vi "mainSC.vi"() -> ()   [LabVIEW 2021]
uses:
  <vilib>/Platform/TimedLoop/XDataNode/timing_clust.ctl
  <vilib>/Platform/TimedLoop/XDataNode/nitl_modes.ctl
  <vilib>/Platform/TimedLoop/XDataNode/wakeup.ctl
  <vilib>/xnet/xnet.llb/XNET Frame CAN.ctl
  <vilib>/xnet/xnet.llb/XNET Frame Type CAN.ctl
  <vilib>/xnet/xnet.llb/XNET Read (Frame CAN).vi
  <vilib>/xnet/xnet.llb/XNET Write (Frame CAN).vi
  <vilib>/Utility/error.llb/Error Cluster From Error Code.vi
  <vilib>/rvi/errors/niLvFpgaAdjustHostInterfaceError.vi
  General Purpose/FPGAref.ctl
  <vilib>/Platform/TimedLoop/XDataNode/XDataNode.xnode
  <vilib>/rvi/interface/nirviMethod/nirviMethod.xnode
  <vilib>/rvi/interface/nirviReadWriteControl/nirviReadWriteControl.xnode
  <vilib>/Platform/TimedLoop/XDataNode/XDNodeRunTimeDep.lvlib
  <vilib>/FPGAPlugInAG/Dynamic/niLvFpga_ReadFifo_Dynamic.vi
  <vilib>/rvi/errors/niLvFpgaMergeErrorWithErrorCode.vi
  NiFpgaLv.dll
  <vilib>/rvi/interface/Simulation/niFpgaSimulationCallBeginRW.vi
panel:
  out "IavFC":dbl
  out "TstackOut":dbl
  out "TstackIn":dbl
  out "FC_ph2":dbl
  out "ErrorBoolean":bool
  out "p_sp_max":dbl
  out "H2_flow":dbl
  in  "AnalogLoopPeriod(ms)":i64=250
  out "q_sp_min":dbl
  out "q_sp_max":dbl
  out "p_sp_min":dbl=2000.0
  out "Con_State 2":u8(ring) items=["Idle"=0, "Busy"=1, "Wait4srcON"=2, "Ready"=3, "VSC mode"=5, "CSC mode"=6, "Error"=9, "Wait4srcOFF"=10, "ISRC mode"=11, "VSRC mode"=12]
  out "ErrorListFCRaw":u8[](array[numeric])
  out "ErrorFC":bool=TRUE
  in  "Main Stop":bool
  in  "Isrc Mode":bool
  in  "Usr Demand":T1(ring)
  in  "Log Influx DB":bool=TRUE
  out "FCPS Voltage [V]":dbl
  out "FCPS Current [A]":dbl
  out "FC Power Setpoint":dbl
  out "Fuel Cell":T2 {"Tstack Out [degC]" format="%.3f"}
  out "Vdc DC Link":dbl
  out "Alarm list":string
  out "Error":u8(ring) items=["None", "Converter (water/temp/desat)", "Overvalue (hardware detected)", "Internal DC bus low", "Internal DC bus high", "External source DC low", "External source DC high", "Grid present (while VSC)", "Grid voltage out of range", "Grid frequency out of range", "No Grid (while CSC)", "Cannot clear (Manual clear needed)", "User Emergency"]
  in  "p_sp":dbl
  in  "q_sp":dbl
  in  "Shutdwn":bool
  in  "Clear":bool
  in  "SEND sp":bool
  in  "Start":bool
  in  "Emergency":bool
  in  "Meas":T3 {"Ia" format="%#.2f"; "Ib" format="%#.2f"; "Ic" format="%#.2f"; "Pa" format="%#.2f"; "Qa" format="%#.2f"; "Va" format="%#.2f"; "Pb" format="%#.2f"; "Qb" format="%#.2f"; "Vb" format="%#.2f"; "Pc" format="%#.2f"; "Qc" format="%#.2f"; "Vc" format="%#.2f"; "P" format="%#.2f"; "Q" format="%#.2f"; "S" format="%#.2f"; "PF" format="%#.2f"; "In" format="%#.2f"; "Vnpe" format="%#.2f"; "Vdc" format="%#.2f"; "Idc" format="%#.2f"; "Pdc" format="%#.2f"}
  out "DC":bool
  out "AC":bool
  out "CAN with Fuel Cell":bool
  out "V_src":dbl
  out "I_src":dbl
  out "Con_State":u8(ring) items=["Idle"=0, "Busy"=1, "Wait4srcON"=2, "Ready"=3, "VSC mode"=5, "CSC mode"=6, "Error"=9, "Wait4srcOFF"=10, "ISRC mode"=11, "VSRC mode"=12]
  in  "Conv CAN [ms]":i64=1
  out "Conv":T4
  out "CAN with Conv":bool
  in  "FC CAN [ms]":i64=50
  out "logging":bool
  in  "Meas [ms]":i64=10
  out "P":dbl format="%#.3f"
  out "Q":dbl format="%#.3f"
  out "S":dbl format="%#.3f"
  out "PF":dbl format="%#.3f"
  out "Measurements":bool
  # "FUEL CELL CONTROL"
  # "CONVERTER CONTROL"
  # "SETPOINTS"
  # "FUEL\nCELL"
  # "DC"
  # "AC"
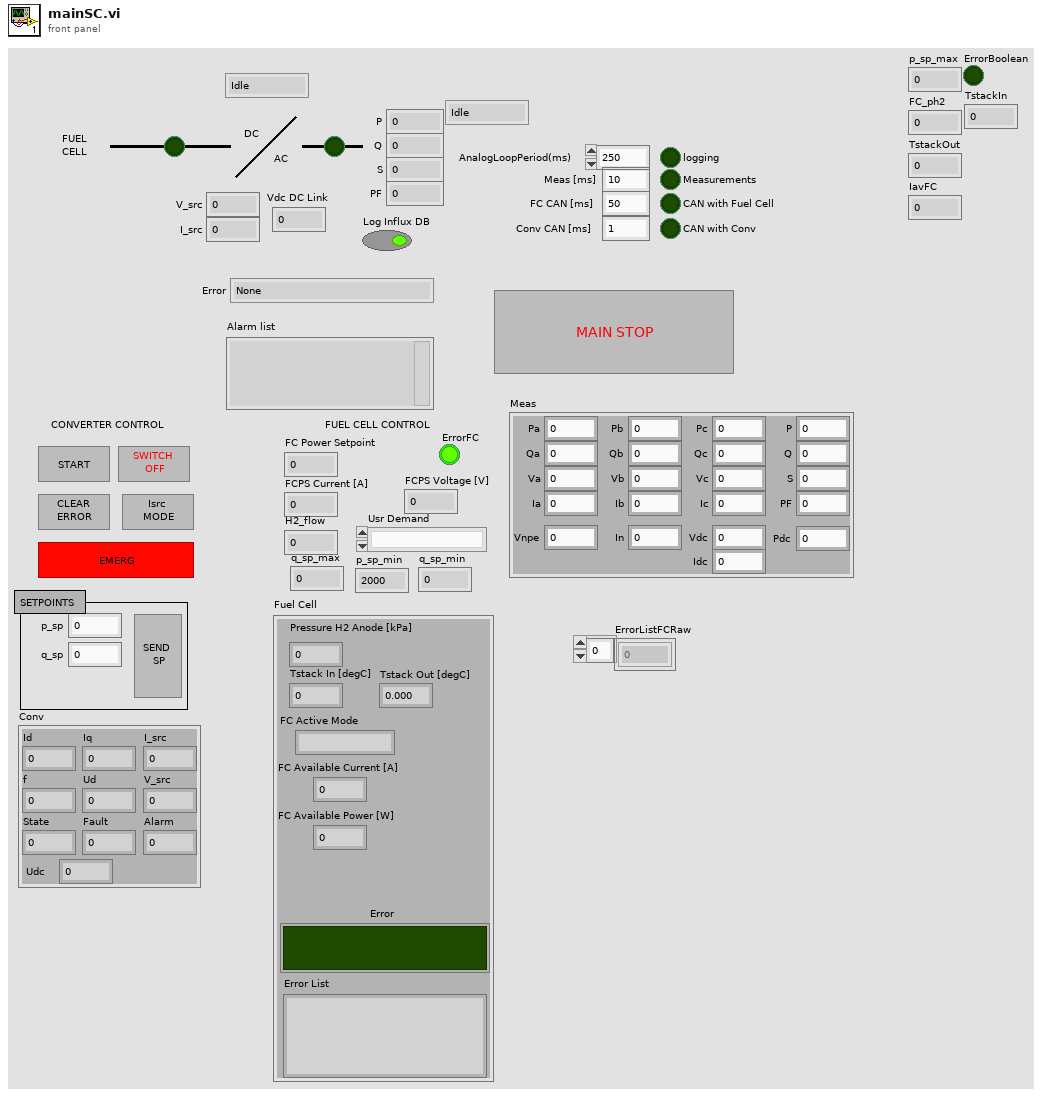
[diagram p1: front panel]
types:
  T1 = enum16{"", "Emergency Shut Down", "Shut Down", "Start"}
  T2 = cluster{"Tstack In [degC]":dbl, "Pressure H2 Anode [kPa]":dbl, "Tstack Out [degC]":dbl, "FC Available Current [A]":dbl, "FC Available Power [W]":dbl, "FC Active Mode":string, "Error":bool, "Error List":string}
  T3 = cluster{"Pa":dbl, "Qa":dbl, "Va":dbl, "Pb":dbl, "Qb":dbl, "Vb":dbl, "Pc":dbl, "Qc":dbl, "Vc":dbl, "P":dbl, "Q":dbl, "S":dbl, "PF":dbl, "In":dbl, "Vnpe":dbl, "Vdc":dbl, "Idc":dbl, "Pdc":dbl, "Ic":dbl, "Ib":dbl, "Ia":dbl}
  T4 = cluster{"Id":dbl, "Iq":dbl, "Ud":dbl, "f":dbl, "I_src":dbl, "V_src":dbl, "State":dbl, "Fault":dbl, "Alarm":dbl, "Udc":dbl}
  T5 = typedef "FPGAref.ctl" = refnum<k20>
  T6 = typedef "XDNodeRunTimeDep.lvlib/timing_clust.ctl" = cluster{"Expected End [f-1]":u64, "Actual End [f-1]":u64, "Finished Late? [f-1]":bool, "Expected End [i-1]":u64, "Actual End [i-1]":u64, "Finished Late? [i-1]":bool, "Expected Start [i]":u64, "Actual Start [i]":u64, "Expected Start [f]":u64, "Actual Start [f]":u64, "Source Name":string, "Structure Name":string, "Period":i64, "Deadline":i64, "Offset":i64, "Start":i64, "Priority":i32, "Timeout":i32, "Mode":T7, "Wakeup Reason":T8, "Error":errorcluster, "Source Type":string, "Secondary Source Type":string, "Global End Time":u64, "Global Start Time":u64, "Frame Duration":u64, "Iteration Duration":u64, "Assigned CPU":i32, "I/O Scan Engine Mode":u32}
  T7 = typedef "XDNodeRunTimeDep.lvlib/nitl_modes.ctl" = enum32{"No Change", "Process missed periods, maintain original phase", "Discard missed periods, maintain original phase", "Process missed periods, ignore original phase", "Discard missed periods, ignore original phase"}
  T8 = typedef "XDNodeRunTimeDep.lvlib/wakeup.ctl" = enum32{"Normal", "Aborted", "Asynchronous wakeup", "Timing source error", "Timed loop error", "Timeout"}
  T9 = typedef "XNET Frame CAN.ctl" = cluster{"timestamp":timestamp, "payload":u8[], "identifier":u32, "type":T10, "extended?":bool, "echo?":bool}
  T10 = typedef "XNET Frame Type CAN.ctl" = u8
  T11 = cluster{"Timestamp":dbl, "P":dbl, "Idc":dbl, "Q":dbl, "Vdc":dbl, "TstackIn":dbl, "Psp":dbl, "Qsp":dbl, "ErrorBoolean":bool, "IavFC":dbl, "p_sp_max":dbl, "StatusConv":u8, "ConnectedFC":bool, "ConnectedGrid":bool, "TstackOut":dbl, "Vdclink":dbl, "FC_ph2":dbl, "p_sp_min":dbl, "q_sp_max":dbl, "q_sp_min":dbl, "FC_po2":dbl, "FCPressure":dbl}
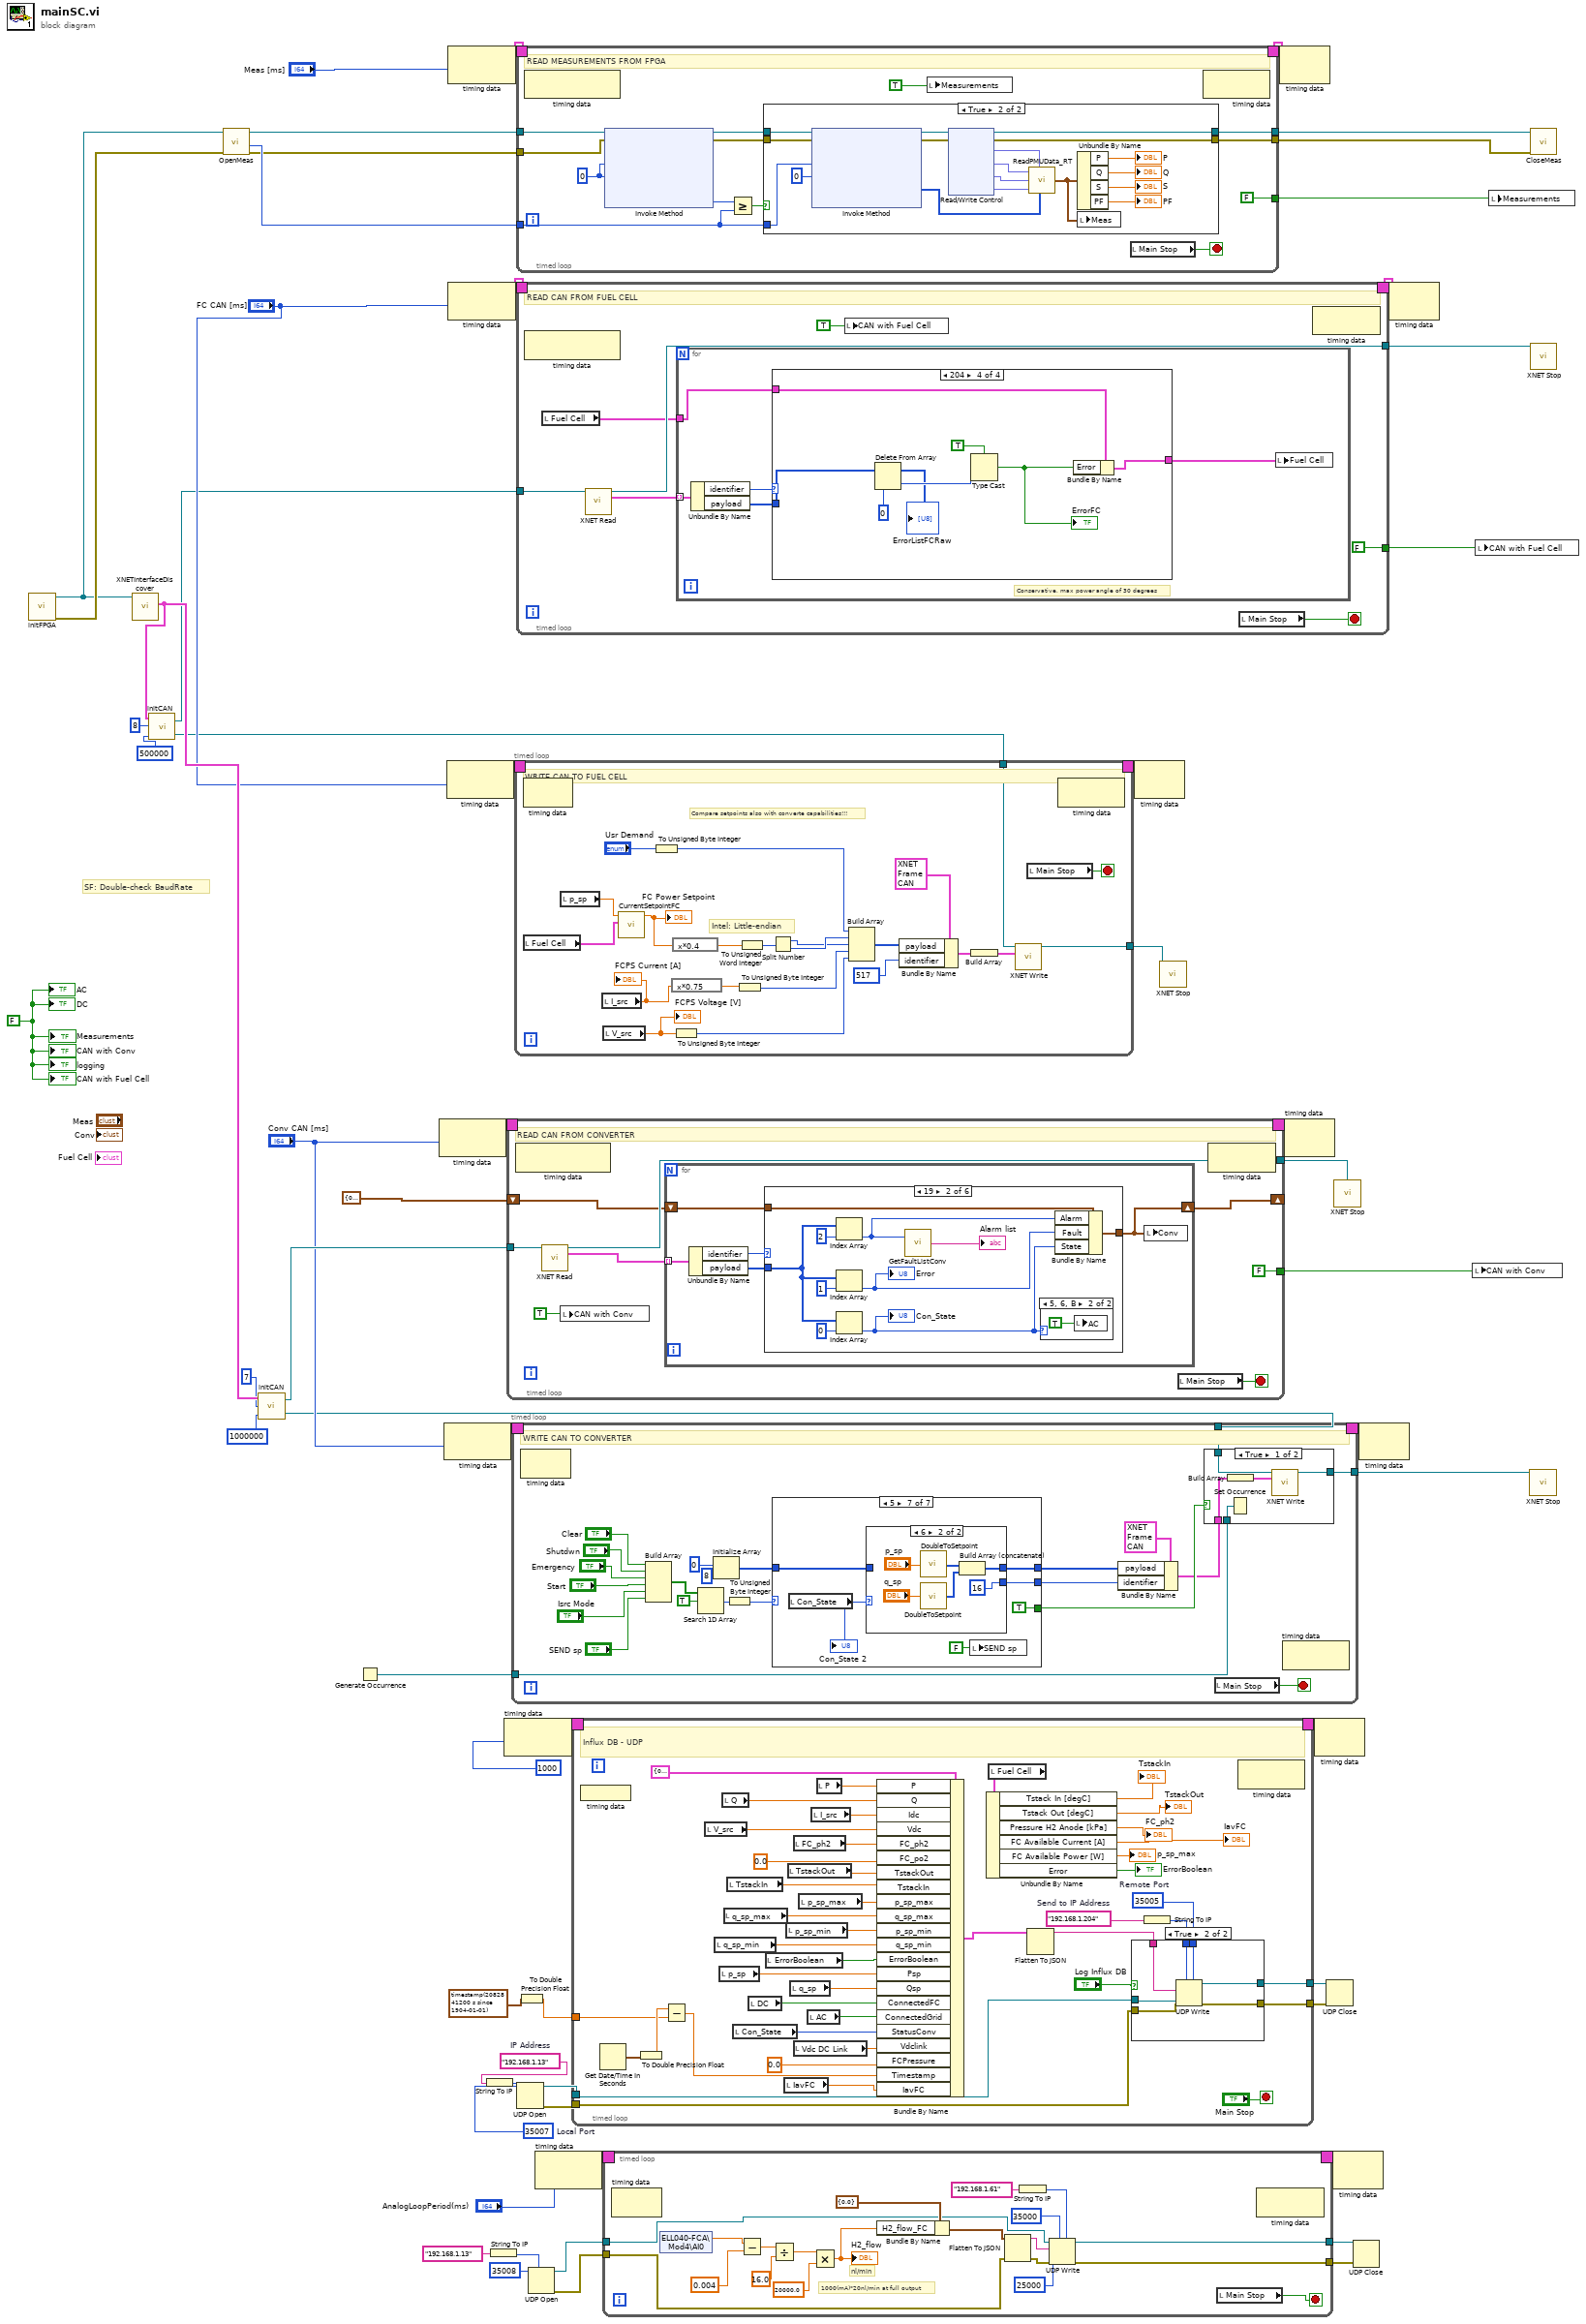
[diagram p0: block diagram]
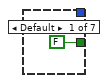
[diagram p5: hidden frame]
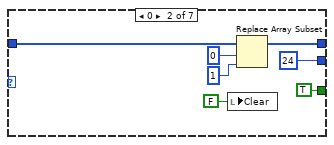
[diagram p6: hidden frame]
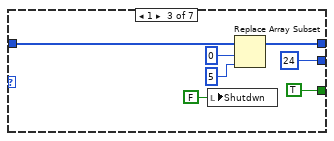
[diagram p7: hidden frame]
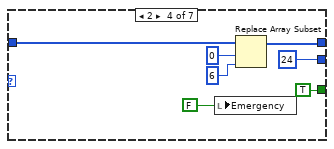
[diagram p8: hidden frame]
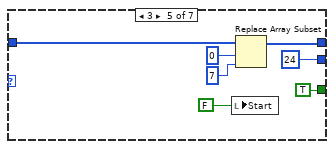
[diagram p9: hidden frame]
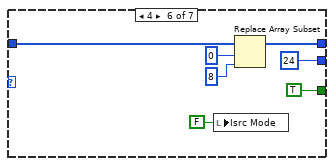
[diagram p10: hidden frame]
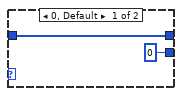
[diagram p11: hidden frame]
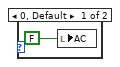
[diagram p13: hidden frame]
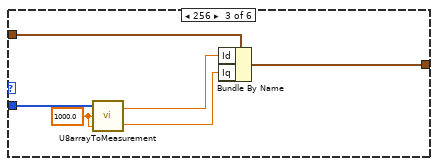
[diagram p14: hidden frame]
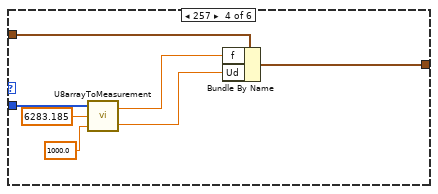
[diagram p15: hidden frame]
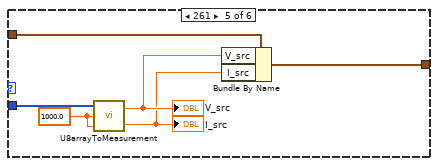
[diagram p16: hidden frame]
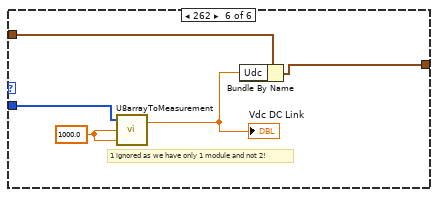
[diagram p17: hidden frame]
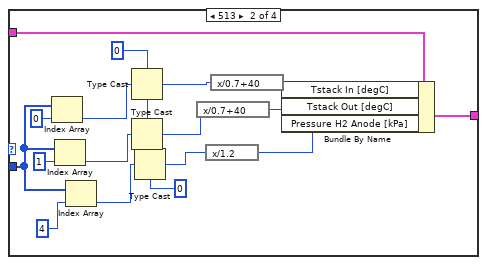
[diagram p19: hidden frame]
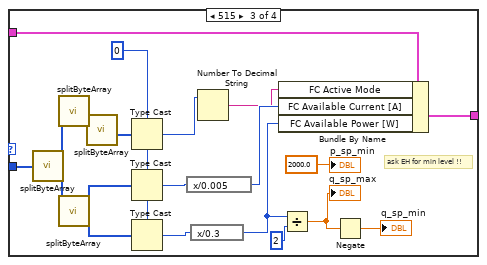
[diagram p20: hidden frame]
diagram:
  w18 = "192.168.1.13"  # IP Address
  w16 = 35007  # Local Port
  w13 = FALSE
  # "SF: Double-check BaudRate"
  n1 = call "initFPGA.vi"() -> ("FPGA VI Reference Out"=w60:T5, "error out"=w61:errorcluster)  [unwired: 4 in]
  n2 = call "XNETInterfaceDiscover.vi"("FPGA in"=w60) -> ("CAN"=w59:cluster{"Interface":refnum<k21>[], "Slot":u32[]})  [unwired: 5 in, 1 out]
  n3 = call "initCAN.vi"("BaudRate"=u32 500000, "SlotNum"=u32 8, "CAN"=w59) -> ("session write"=w35:refnum<k21>, "session read"=w34:refnum<k21>)
  n4 = call "OpenMeas.vi"("error in"=w61, "FPGA in"=w60) -> ("error out"=w26:errorcluster, "Nsamples"=w30:u32, "FPGA out"=w31:T5)  [unwired: 7 in]
  n5 = call "initCAN.vi"("BaudRate"=u32 1000000, "SlotNum"=u32 7, "CAN"=w59) -> ("session write"=w36:refnum<k21>, "session read"=w42:refnum<k21>)
  n6 = Generate Occurrence() -> (w55:refnum<k4>)
  n7 = node-c288("Conv CAN [ms]") -> (w50:T6)
  n8 = node-c288("Conv CAN [ms]") -> (w48:T6)
  n9 = node-c288("FC CAN [ms]") -> (w52:T6)
  n10 = node-c288("Meas [ms]") -> (w33:T6)
  n11 = node-c288("FC CAN [ms]") -> (w54:T6)
  n12 = String To IP(1:w18) -> (0:w17:u32)
  n13 = String To IP(1:"192.168.1.13" ("name")) -> (0:w3:u32)
  n14 = node-c288(1000) -> (w23:T6)
  n15 = timed-loop {
    timing: w50 -> [_]
    timing-out: [_] -> w49
    tunnel: w42 -> [w69]
    tunnel: [w67] -> w44
    shift-right: [w66] -> _
    shift-left: T4 {"Id"=0.0, "Iq"=0.0, "Ud"=328.594, "f"=49.93629823091314, "I_src"=-0.481, "V_src"=252.498, "State"=0.0, "Fault"=0.0, "Alarm"=0.0, "Udc"=0.0} ("Conv") -> [w65]
    tunnel: [FALSE ("stop CAN")] -> w39
    stop <- w64 stop-if-true
    # "READ CAN FROM CONVERTER"
    n16 = node-c288() -> ()  [unwired: 1 in, 1 out]
    n17 = call-poly <vilib>:"XNET Read.vi"("session in"=w69) -> ("session out"=w67:refnum<k21>, "data"=w68:T9[])  [unwired: 11 in, 2 out]
    n18 = local write "CAN with Conv"(TRUE) -> ()
    n19 = for {
      tunnel: w68 -> [w72] mode=indexing
      shift-right: [w70] -> w66
      shift-left: w65 -> [w71]
      n20 = Unbundle By Name(w72) -> ("identifier"=w74:u32, "payload"=w73:u8[])
      n21 = case shown="19" w74 {
        tunnel: w73 -> [_ w79 w93 w100 w106 w110]
        tunnel: w71 -> [w75 w82 w91 w97 w103 w108]
        tunnel: [w75 w81 w88 w96 w104 w109] -> w70
        frame 0, Default {
        }
        frame 25 {
          n22 = Index Array(array=w79, index=2) -> (element=w77:u8)
          n23 = Index Array(array=w79, index=1) -> (element=w78:u8)
          "Error" <- w78
          n24 = Index Array(array=w79, index=0) -> (element=w80:u8)
          "Con_State" <- w80
          n25 = call "GetFaultListConv.vi"("Fault message"=w77) -> ("Fault list"=→"Alarm list":string)  [unwired: 1 in]
          n26 = case shown="5, 6, B" w80 {
            frame 0, Default {
              n27 = local write "AC"(FALSE) -> ()
            }
            frame 5, 6, 11 {
              n28 = local write "AC"(TRUE) -> ()
            }
          }
          n29 = Bundle By Name(cluster=w82, "Alarm"=w77, "Fault"=w78, "State"=w80) -> (w81:T4)
        }
        frame 256 {
          w92 = 1000.0 ("factor 1")
          n30 = call "U8arrayToMeasurement.vi"("factor 2"=w92, "factor 1"=w92, "payload"=w93) -> ("Meas 2"=w89:dbl, "Meas 1"=w90:dbl)
          n31 = Bundle By Name(cluster=w91, "Id"=w90, "Iq"=w89) -> (w88:T4)
        }
        frame 257 {
          n32 = call "U8arrayToMeasurement.vi"("factor 2"=1000.0 ("factor 1"), "factor 1"=6283.185 ("factor 2"), "payload"=w100) -> ("Meas 2"=w98:dbl, "Meas 1"=w99:dbl)
          n33 = Bundle By Name(cluster=w97, "f"=w99, "Ud"=w98) -> (w96:T4)
        }
        frame 261 {
          w105 = 1000.0 ("factor 1")
          n34 = call "U8arrayToMeasurement.vi"("factor 2"=w105, "factor 1"=w105, "payload"=w106) -> ("Meas 2"=w101:dbl, "Meas 1"=w102:dbl)
          "V_src" <- w102
          "I_src" <- w101
          n35 = Bundle By Name(cluster=w103, "V_src"=w102, "I_src"=w101) -> (w104:T4)
        }
        frame 262 {
          w111 = 1000.0 ("factor 1")
          # "1 ignored as we have only 1 module and not 2!"
          n36 = call "U8arrayToMeasurement.vi"("factor 2"=w111, "factor 1"=w111, "payload"=w110) -> ("Meas 1"=w107:dbl)  [unwired: 1 out]
          "Vdc DC Link" <- w107
          n37 = Bundle By Name(cluster=w108, "Udc"=w107) -> (w109:T4)
        }
      }
      n38 = local write "Conv"(w70) -> ()
    }
    n39 = local read "Main Stop"() -> (w64:bool)
    n40 = node-c288() -> ()  [unwired: 1 in, 1 out]
  }
  n41 = timed-loop {
    tunnel: w36 -> [w127]
    tunnel: [w126] -> w38
    timing: w48 -> [_]
    timing-out: [_] -> w47
    tunnel: w55 -> [w115]
    stop <- w125 stop-if-true
    # "WRITE CAN TO CONVERTER"
    n42 = node-c288() -> ()  [unwired: 1 in, 1 out]
    n43 = Build Array("Clear", "Shutdwn", "Emergency", "Start", "Isrc Mode", "SEND sp") -> (w124:bool[])
    n44 = Search 1D Array(1D array=w124, element=TRUE) -> (index of element=w116:i32)  [unwired: 1 in]
    n45 = Initialize Array(u8 0, 8 ("dimension size")) -> (w133:u8[])
    n46 = To Unsigned Byte Integer(number=w116) -> (unsigned 8bit integer=w122:u8)
    n47 = case shown="5" w122 {
      tunnel: [_ w149 w156 w162 w169 w177 w184] -> w132
      tunnel: [_ u32 24 ("identifier") u32 24 ("identifier") u32 24 ("identifier") u32 24 ("identifier") u32 24 ("identifier") w181] -> w131
      tunnel: w133 -> [_ w147 w155 w163 w170 w176 w179]
      tunnel: [FALSE TRUE TRUE TRUE TRUE TRUE TRUE] -> w129
      frame Default {
      }
      frame 0 {
        n48 = local write "Clear"(FALSE ("Clear")) -> ()
        n49 = Replace Array Subset(array=w147, new element=u8 1 ("new element/subarray"), index=0) -> (w149:u8[])
      }
      frame 1 {
        n50 = local write "Shutdwn"(FALSE ("Shutdwn")) -> ()
        n51 = Replace Array Subset(array=w155, new element=u8 5 ("new element/subarray"), index=0) -> (w156:u8[])
      }
      frame 2 {
        n52 = local write "Emergency"(FALSE ("Idc cmd")) -> ()
        n53 = Replace Array Subset(array=w163, new element=u8 6 ("new element/subarray"), index=0) -> (w162:u8[])
      }
      frame 3 {
        n54 = local write "Start"(FALSE ("Idc cmd")) -> ()
        n55 = Replace Array Subset(array=w170, new element=u8 7 ("new element/subarray"), index=0) -> (w169:u8[])
      }
      frame 4 {
        n56 = local write "Isrc Mode"(FALSE ("Isrc Mode")) -> ()
        n57 = Replace Array Subset(array=w176, new element=u8 8 ("new element/subarray"), index=0) -> (w177:u8[])
      }
      frame 5 {
        n58 = local read "Con_State"() -> (w180:u8)
        "Con_State 2" <- w180
        n59 = case shown="6" w180 {
          tunnel: [w186 w188] -> w184
          tunnel: [u32 0 ("identifier") u32 16 ("identifier")] -> w181
          tunnel: w179 -> [w186 _]
          frame 0, Default {
          }
          frame 6 {
            n60 = call "DoubleToSetpoint.vi"("Double"="p_sp") -> ("SP"=w189:u8[])
            n61 = call "DoubleToSetpoint.vi"("Double"="q_sp") -> ("SP"=w190:u8[])
            n62 = Build Array (concatenate)(w189, w190) -> (w188:u8[])
          }
        }
        n63 = local write "SEND sp"(FALSE ("SEND sp")) -> ()
      }
    }
    n64 = Bundle By Name(cluster=T9 {"timestamp"=timestamp(0 s since 1904-01-01), "payload"=[], "identifier"=0, "type"=0, "extended?"=FALSE, "echo?"=FALSE} ("CAN frame 3"), "payload"=w132, "identifier"=w131) -> (w128:T9)
    n65 = case shown="True" w129 {
      tunnel: w128 -> [w142 _]
      tunnel: w127 -> [w140 _]
      tunnel: [w139 _] -> w126
      tunnel: w115 -> [w138 _]
      frame True {
        n66 = Build Array(w142) -> (w141:T9[])
        n67 = Set Occurrence(w138) -> ()
        n68 = call-poly <vilib>:"XNET Write.vi"("session in"=w140, "data"=w141) -> ("session out"=w139:refnum<k21>)  [unwired: 12 in, 1 out]
      }
      frame False {
      }
    }
    n69 = local read "Main Stop"() -> (w125:bool)
    n70 = node-c288() -> ()  [unwired: 1 in, 1 out]
  }
  n71 = timed-loop {
    timing: w52 -> [_]
    timing-out: [_] -> w51
    tunnel: w35 -> [w209]
    tunnel: [w207] -> w46
    stop <- w208 stop-if-true
    # "Compare setpoints also with converte capabilities!!!"
    # "Intel: Little-endian"
    # "WRITE CAN TO FUEL CELL"
    n72 = node-c288() -> ()  [unwired: 1 in, 1 out]
    n73 = local read "Fuel Cell"() -> (w193:T2)
    n74 = local read "p_sp"() -> (w195:dbl)
    n75 = local read "I_src"() -> (w197:dbl)
    "FCPS Current [A]" <- w197
    n76 = local read "V_src"() -> (w196:dbl)
    "FCPS Voltage [V]" <- w196
    n77 = call "CurrentSetpointFC.vi"("Fuel Cell"=w193, "p_sp"=w195) -> ("P_sp_FC"=w194:dbl)  [unwired: 9 in]
    "FC Power Setpoint" <- w194
    n78 = To Unsigned Byte Integer(number="Usr Demand") -> (unsigned 8bit integer=w198:u8)
    n79 = expression code="x*0.75"(w197) -> (w206:dbl)
    n80 = expression code="x*0.4"(w194) -> (w205:dbl)
    n81 = To Unsigned Byte Integer(number=w196) -> (unsigned 8bit integer=w203:u8)
    n82 = To Unsigned Byte Integer(number=w206) -> (unsigned 8bit integer=w202:u8)
    n83 = To Unsigned Word Integer(number=w205) -> (unsigned 16bit integer=w204:u16)
    n84 = Split Number(x=w204) -> (hi(x)=w200:u8, lo(x)=w201:u8)
    n85 = Build Array(w198, w201, w200, w202, w203) -> (w214:u8[])
    n86 = Bundle By Name(cluster=T9 {"timestamp"=timestamp(0 s since 1904-01-01), "payload"=[], "identifier"=0, "type"=0, "extended?"=FALSE, "echo?"=FALSE} ("CAN frame 3"), "payload"=w214, "identifier"=u32 517) -> (w211:T9)
    n87 = Build Array(w211) -> (w210:T9[])
    n88 = call-poly <vilib>:"XNET Write.vi"("session in"=w209, "data"=w210) -> ("session out"=w207:refnum<k21>)  [unwired: 12 in, 1 out]
    n89 = local read "Main Stop"() -> (w208:bool)
    n90 = node-c288() -> ()  [unwired: 1 in, 1 out]
  }
  n91 = timed-loop {
    timing: w33 -> [_]
    timing-out: [_] -> w32
    tunnel: w31 -> [w224]
    tunnel: [w229] -> w27
    tunnel: [w228] -> w29
    tunnel: w30 -> [w218]
    tunnel: [FALSE] -> w28
    tunnel: w26 -> [w222]
    stop <- w226 stop-if-true
    w217 = 0 ("Timeout (ms)")
    # "READ MEASUREMENTS FROM FPGA"
    n92 = node-c288() -> ()  [unwired: 1 in, 1 out]
    n93 = xnode "Invoke Method"("FPGA VI Reference In"=w224, "error in"=w222, "Number of Elements"=w217, "Timeout (ms)"=w217) -> ("FPGA VI Reference Out"=w223:T5, "error out"=w221:errorcluster, "Elements Remaining"=w219:u32)  [unwired: 1 out]
    n94 = Greater Or Equal?(x=w219, y=w218) -> (x >= y?=w220:bool)
    n95 = case shown="True" w220 {
      tunnel: [w231 w239] -> w229
      tunnel: [w230 w238] -> w228
      tunnel: w223 -> [w231 w244]
      tunnel: w221 -> [w230 w243]
      tunnel: w218 -> [_ w242]
      frame False {
      }
      frame True {
        n96 = xnode "Invoke Method"("FPGA VI Reference In"=w244, "error in"=w243, "Number of Elements"=w242, "Timeout (ms)"=0) -> ("FPGA VI Reference Out"=w241:T5, "error out"=w240:errorcluster, "Data"=w237:u32[])  [unwired: 1 out]
        n97 = xnode "Read/Write Control"("FPGA VI Reference In"=w241, "error in"=w240) -> ("FPGA VI Reference Out"=w239:T5, "error out"=w238:errorcluster, "Vnpe"=w233:fxp<+,20,5>, "In"=w234:fxp<+,20,5>, "Vdc"=w235:fxp<+/-,20,5>, "Idc"=w236:fxp<+/-,20,5>)
        n98 = call "ReadPMUData_RT.vi"("In"=w234, "Vnpe"=w233, "Vdc"=w235, "Idc"=w236, "data in"=w237) -> ("proc_meas"=w232:T3)
        n99 = Unbundle By Name(w232) -> ("P"=→"P":dbl, "Q"=→"Q":dbl, "S"=→"S":dbl, "PF"=→"PF":dbl)
        n100 = local write "Meas"(w232) -> ()
      }
    }
    n101 = local write "Measurements"(TRUE) -> ()
    n102 = local read "Main Stop"() -> (w226:bool)
    n103 = node-c288() -> ()  [unwired: 1 in, 1 out]
  }
  n104 = timed-loop {
    timing: w54 -> [_]
    timing-out: [_] -> w53
    tunnel: w34 -> [w256]
    tunnel: [w255] -> w43
    tunnel: [FALSE ("CAN with Fuel Cell")] -> w41
    stop <- w258 stop-if-true
    # "READ CAN FROM FUEL CELL"
    n105 = node-c288() -> ()  [unwired: 1 in, 1 out]
    n106 = local read "Fuel Cell"() -> (w252:T2)
    n107 = call-poly <vilib>:"XNET Read.vi"("session in"=w256) -> ("session out"=w255:refnum<k21>, "data"=w257:T9[])  [unwired: 11 in, 2 out]
    n108 = for {
      tunnel: w257 -> [w262] mode=indexing
      tunnel: w252 -> [w259]
      # "Conservative, max power angle of 30 degrees"
      n109 = Unbundle By Name(w262) -> ("identifier"=w263:u32, "payload"=w261:u8[])
      n110 = case shown="204" w263 {
        tunnel: w261 -> [_ w274 w296 w307]
        tunnel: w259 -> [w264 w279 w300 w309]
        tunnel: [w264 w278 w299 w308] -> w260
        frame 0, Default {
        }
        frame 513 {
          w281 = u16 0
          n111 = Index Array(array=w274, index=0) -> (element=w276:u8)
          n112 = Index Array(array=w274, index=1) -> (element=w272:u8)
          n113 = Index Array(array=w274, index=4) -> (element=w271:u8)
          n114 = Type Cast(type=w281, x=w276) -> (*(type *) &x=w270:u16)
          n115 = Type Cast(type=w281, x=w272) -> (*(type *) &x=w269:u16)
          n116 = Type Cast(type=i16 0, x=w271) -> (*(type *) &x=w268:i16)
          n117 = expression code="x/0.7+40"(w269) -> (w266:u16)
          n118 = expression code="x/1.2"(w268) -> (w265:i16)
          n119 = expression code="x/0.7+40"(w270) -> (w267:u16)
          n120 = Bundle By Name(cluster=w279, "Tstack In [degC]"=w267, "Tstack Out [degC]"=w266, "Pressure H2 Anode [kPa]"=w265) -> (w278:T2)
        }
        frame 515 {
          w301 = u16 0
          # "ask EH for min level !!"
          n121 = call "splitByteArray.vi"("array"=w296) -> ("first half"=w298:u8[], "second half"=w297:u8[])  [unwired: 4 in]
          n122 = call "splitByteArray.vi"("array"=w298) -> ("second half"=w293:u8[])  [unwired: 4 in, 1 out]
          n123 = call "splitByteArray.vi"("array"=w297) -> ("first half"=w295:u8[], "second half"=w294:u8[])  [unwired: 4 in]
          n124 = call "splitByteArray.vi"("array"=w293) -> ("second half"=w292:u8[])  [unwired: 4 in, 1 out]
          n125 = Type Cast(type=w301, x=w292) -> (*(type *) &x=w288:u16)
          n126 = Type Cast(type=w301, x=w295) -> (*(type *) &x=w291:u16)
          n127 = Type Cast(type=w301, x=w294) -> (*(type *) &x=w289:u16)
          n128 = expression code="x/0.005"(w291) -> (w290:u16)
          n129 = expression code="x/0.3"(w289) -> (w285:u16)
          n130 = Number To Decimal String(number=w288) -> (decimal integer string=w287:string)  [unwired: 1 in]
          n131 = Bundle By Name(cluster=w300, "FC Active Mode"=w287, "FC Available Current [A]"=w290, "FC Available Power [W]"=w285) -> (w299:T2)
          n132 = Divide(x=w285, y=u16 2) -> (x/y=w283:dbl)
          "q_sp_max" <- w283
          n133 = Negate(x=w283) -> (-x=→"q_sp_min":dbl)
          "p_sp_min" <- 2000.0
        }
        frame 516 {
          n134 = Delete From Array(array=w307, index=0) -> (deleted portion=w305:u8, array with subset deleted=→"ErrorListFCRaw":u8[])  [unwired: 1 in]
          n135 = Type Cast(type=TRUE, x=w305) -> (*(type *) &x=w302:bool)
          "ErrorFC" <- w302
          n136 = Bundle By Name(cluster=w309, "Error"=w302) -> (w308:T2)
        }
      }
      n137 = local write "Fuel Cell"(w260) -> ()
    }
    n138 = local write "CAN with Fuel Cell"(TRUE ("CAN with Fuel Cell")) -> ()
    n139 = local read "Main Stop"() -> (w258:bool)
    n140 = node-c288() -> ()  [unwired: 1 in, 1 out]
  }
  n141 = UDP Open(7:w17, 11:w16) -> (port=w19:refnum<k16>, 0:w20:errorcluster)  [unwired: 3 in, 1 out]
  n142 = To Double Precision Float(number=timestamp(2082841200 s since 1904-01-01)) -> (double precision float=w11:dbl)
  n143 = UDP Open(7:w3, 11:u16 35008 ("port")) -> (port=w4:refnum<k16>, 0:w5:errorcluster)  [unwired: 3 in, 1 out]
  n144 = node-c288("AnalogLoopPeriod(ms)") -> (w10:T6)
  n145 = timed-loop "Timed Loop" {
    timing: w23 -> [_]
    timing-out: [_] -> w22
    tunnel: w20 -> [w354]
    tunnel: w19 -> [w353]
    tunnel: [w352] -> w15
    tunnel: [w349] -> w14
    tunnel: w11 -> [w344]
    stop <- "Main Stop" stop-if-true
    w317 = "192.168.1.204"  # Send to IP Address
    w315 = 35005  # Remote Port
    # "Influx DB - UDP"
    n146 = node-c288() -> ()  [unwired: 1 in]
    n147 = Get Date/Time In Seconds() -> (seconds since 1Jan1904=w346:timestamp)
    n148 = To Double Precision Float(number=w346) -> (double precision float=w345:dbl)
    n149 = Subtract(x=w345, y=w344) -> (x-y=w318:dbl)
    n150 = local read "V_src"() -> (w341:dbl)
    n151 = local read "q_sp_min"() -> (w327:dbl)
    n152 = local read "p_sp"() -> (w325:dbl)
    n153 = local read "Q"() -> (w342:dbl)
    n154 = local read "q_sp_max"() -> (w329:dbl)
    n155 = local read "TstackIn"() -> (w332:dbl)
    n156 = local read "Con_State"() -> (w321:u8)
    n157 = local read "DC"() -> (w323:bool)
    n158 = local read "ErrorBoolean"() -> (w326:bool)
    n159 = local read "IavFC"() -> (w312:dbl)
    n160 = local read "p_sp_min"() -> (w328:dbl)
    n161 = local read "TstackOut"() -> (w331:dbl)
    n162 = local read "q_sp"() -> (w324:dbl)
    n163 = local read "FC_ph2"() -> (w337:dbl)
    n164 = local read "Vdc DC Link"() -> (w320:dbl)
    n165 = local read "p_sp_max"() -> (w330:dbl)
    n166 = local read "AC"() -> (w322:bool)
    n167 = local read "I_src"() -> (w343:dbl)
    n168 = local read "P"() -> (w339:dbl)
    n169 = Bundle By Name(cluster=T11 {"Timestamp"=0.0, "P"=0.0, "Idc"=0.0, "Q"=0.0, "Vdc"=0.0, "TstackIn"=0.0, "Psp"=0.0, "Qsp"=0.0, "ErrorBoolean"=FALSE, "IavFC"=0.0, "p_sp_max"=0.0, "StatusConv"=0, "ConnectedFC"=TRUE, "ConnectedGrid"=TRUE, "TstackOut"=0.0, "Vdclink"=0.0, "FC_ph2"=0.0, "p_sp_min"=0.0, "q_sp_max"=0.0, "q_sp_min"=0.0, "FC_po2"=0.0, "FCPressure"=0.0} ("input cluster"), "P"=w339, "Q"=w342, "Idc"=w343, "Vdc"=w341, "FC_ph2"=w337, "FC_po2"=0.0, "TstackOut"=w331, "TstackIn"=w332, "p_sp_max"=w330, "q_sp_max"=w329, "p_sp_min"=w328, "q_sp_min"=w327, "ErrorBoolean"=w326, "Psp"=w325, "Qsp"=w324, "ConnectedFC"=w323, "ConnectedGrid"=w322, "StatusConv"=w321, "Vdclink"=w320, "FCPressure"=0.0, "Timestamp"=w318, "IavFC"=w312) -> (w351:T11)
    n170 = local read "Fuel Cell"() -> (w348:T2)
    n171 = Unbundle By Name(w348) -> ("Tstack In [degC]"=→"TstackIn":dbl, "Tstack Out [degC]"=→"TstackOut":dbl, "Pressure H2 Anode [kPa]"=→"FC_ph2":dbl, "FC Available Current [A]"=→"IavFC":dbl, "FC Available Power [W]"=→"p_sp_max":dbl, "Error"=→"ErrorBoolean":bool)
    n172 = Flatten To JSON(anything=w351) -> (JSON string=w355:string)  [unwired: 2 in, 1 out]
    n173 = String To IP(1:w317) -> (0:w316:u32)
    n174 = case shown="True" "Log Influx DB" {
      tunnel: w355 -> [_ w363]
      tunnel: w354 -> [w356 w362]
      tunnel: w353 -> [w357 w364]
      tunnel: [w357 w361] -> w352
      tunnel: [w356 w360] -> w349
      tunnel: w316 -> [_ w359]
      tunnel: w315 -> [_ w358]
      frame False {
      }
      frame True {
        n175 = UDP Write(address=w359, port or service name=w358, connection ID=w364, data in=w363, 8:w362) -> (error out=w360:errorcluster, 3:w361:refnum<k16>)  [unwired: 1 in]
      }
    }
    n176 = node-c288() -> ()  [unwired: 1 in, 1 out]
  }
  n177 = timed-loop {
    timing: w10 -> [_]
    timing-out: [_] -> w9
    tunnel: [w380] -> w7
    tunnel: [w379] -> w6
    tunnel: w5 -> [w373]
    tunnel: w4 -> [w368]
    stop <- w367 stop-if-true
    # "nl/min"
    # "1000(mA)*20nl/min at full output"
    n178 = node-c288() -> ()  [unwired: 1 in, 1 out]
    n179 = shared-variable "ELL040-FCA\\Mod4\\AI0"() -> (w386:dbl)  [unwired: 1 in, 1 out]
    n180 = Subtract(x=w386, y=0.004) -> (x-y=w384:dbl)
    n181 = Divide(x=w384, y=16.0) -> (x/y=w382:dbl)
    n182 = Multiply(x=w382, y=20000.0) -> (x*y=w377:dbl)
    "H2_flow" <- w377
    n183 = Bundle By Name(cluster=cluster{"H2_flow_FC":dbl} {"H2_flow_FC"=0.0}, "H2_flow_FC"=w377) -> (w374:cluster{"H2_flow_FC":dbl})
    n184 = Flatten To JSON(anything=w374, error in (no error)=w373) -> (JSON string=w376:string, 11:w375:errorcluster)  [unwired: 1 in]
    n185 = String To IP(1:"192.168.1.61" ("name")) -> (0:w369:u32)
    n186 = UDP Write(address=u32 35000, port or service name=w369, connection ID=w368, data in=w376, 8:w375, 9:25000 ("timeout ms (25000)")) -> (error out=w379:errorcluster, 3:w380:refnum<k16>)
    n187 = local read "Main Stop"() -> (w367:bool)
    n188 = node-c288() -> ()  [unwired: 1 in, 1 out]
  }
  n189 = node-c288(w51) -> ()  [unwired: 1 out]
  n190 = call <vilib>:"XNET Stop.vi"("session in"=w46) -> ()  [unwired: 13 in, 2 out]
  n191 = node-c288(w32) -> ()  [unwired: 1 out]
  n192 = node-c288(w49) -> ()  [unwired: 1 out]
  n193 = node-c288(w22) -> ()  [unwired: 1 out]
  n194 = UDP Close(connection ID=w15, 8:w14) -> ()  [unwired: 2 out]
  n195 = node-c288(w9) -> ()  [unwired: 1 out]
  n196 = call <vilib>:"XNET Stop.vi"("session in"=w44) -> ()  [unwired: 13 in, 2 out]
  n197 = UDP Close(connection ID=w7, 8:w6) -> ()  [unwired: 2 out]
  n198 = node-c288(w47) -> ()  [unwired: 1 out]
  n199 = node-c288(w53) -> ()  [unwired: 1 out]
  n200 = local write "CAN with Conv"(w39) -> ()
  n201 = local write "CAN with Fuel Cell"(w41) -> ()
  n202 = local write "Measurements"(w28) -> ()
  n203 = call <vilib>:"XNET Stop.vi"("session in"=w38) -> ()  [unwired: 13 in, 2 out]
  n204 = call "CloseMeas.vi"("error in (no error)"=w29, "FPGA in"=w27) -> ()  [unwired: 10 in]
  n205 = call <vilib>:"XNET Stop.vi"("session in"=w43) -> ()  [unwired: 13 in, 2 out]
  "Measurements" <- w13
  "logging" <- w13
  "DC" <- w13
  "CAN with Conv" <- w13
  "AC" <- w13
  "CAN with Fuel Cell" <- w13
